vi "Test Engine Actor Register Events.vi"(8 "error in (no error)":errorcluster, 9 "Registrant Address":refnum<class "Message Enqueuer.lvclass">, 10 "Event Source Address":refnum<class "Message Enqueuer.lvclass">, 11 "TestBench in":refnum<class "TestBench.lvclass">) -> (0 "error out":errorcluster, 3 "TestBench out":refnum<class "TestBench.lvclass">)   [LabVIEW 2019, in "TestBench.lvlib" / "TestBench.lvclass"]
uses:
  TestBench.lvclass
  <vilib>/ActorFramework/Message Enqueuer/Message Enqueuer.lvclass
  TestEngine/TestEngine/TestEngineReference.lvclass
  C:/Program Files (x86)/National Instruments/LabVIEW 2019/vi.lib/NI/Event Source Actor/Event Source/Event/Event.lvclass
  TestBench Messages/Insert VI Msg/Insert VI Msg.lvclass
  C:/Program Files (x86)/National Instruments/LabVIEW 2019/vi.lib/NI/Event Source Actor/Event Source/Event Source Messages/Event Generated Msg/Event Generated Msg.lvclass
  TestBench Messages/Write DetailedResult Msg/Write DetailedResult Msg.lvclass
  TestEngine/TestEngine/TestResultInformation.lvclass
  TestBench Messages/Write TestResultInformation Msg/Write TestResultInformation Msg.lvclass
  TestEngine/TestEngine/Number of Steps.lvclass
  TestBench Messages/SetSlide Msg/SetSlide Msg.lvclass
  TestEngine/TestEngine/TestDetailedResult.lvclass
  TestBench Messages/StepCount Msg/StepCount Msg.lvclass
  <vilib>/NI/Event Source Actor/Event Source/Event/Event.lvclass/Event.ctl
  <vilib>/NI/Event Source Actor/Event Source/Event Source Messages/Register Msg/Register Msg.lvclass/Register Msg.ctl
  <vilib>/ActorFramework/Message Enqueuer/Message Enqueuer.lvclass/Message Enqueuer.ctl
  <vilib>/ActorFramework/Message Enqueuer/Enqueue.vi
  <vilib>/NI/Event Source Actor/Event Source/Event Source Messages/Register Msg/Register Msg.lvclass
  C:/Program Files (x86)/National Instruments/LabVIEW 2019/vi.lib/ActorFramework/Message/Message.lvclass
  <vilib>/ActorFramework/Message Priority Queue/Priority Enqueue.vi
  <vilib>/NI/Event Source Actor/Event Source/Event/Event.lvclass
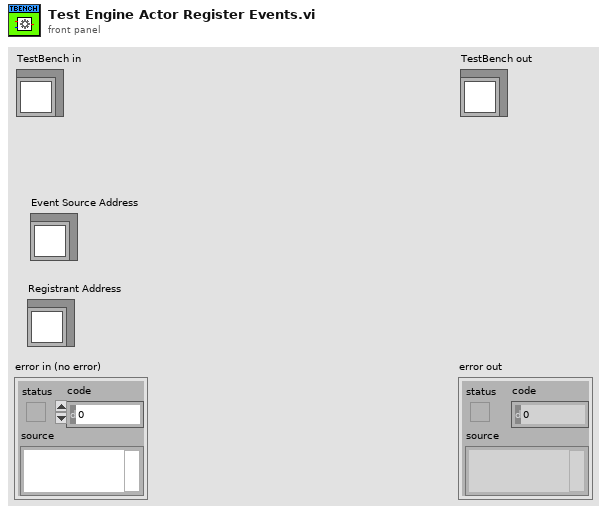
[diagram p1: front panel]
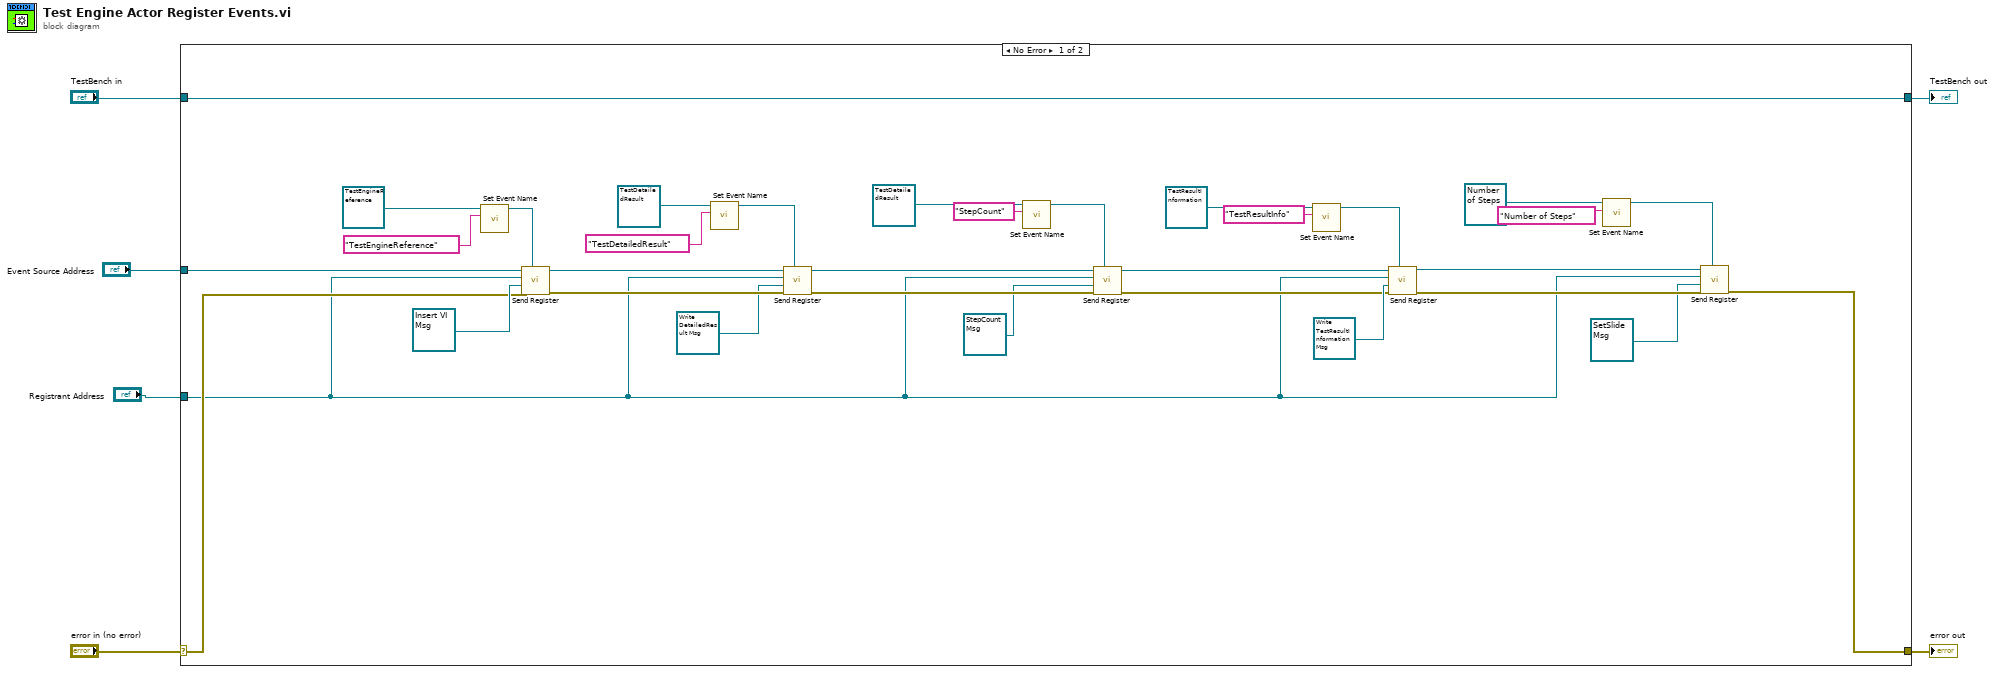
[diagram p0: block diagram]
diagram:
  n1 = case shown="No Error" "error in (no error)" {
    selector: "error in (no error)" -> [w10 w41]
    tunnel: [w7 w41] -> w5
    tunnel: [w39 w40] -> w3
    tunnel: "TestBench in" -> [w39 w40]
    tunnel: "Registrant Address" -> [w9 _]
    tunnel: "Event Source Address" -> [w8 _]
    frame No Error {
      n2 = call <vilib>:"Set Event Name.vi"("Name (Generic)"="TestEngineReference" ("ActorCoreEventMassage"), "Event In"=refnum<class "TestEngineReference.lvclass"> refnum ("TestEngine.lvlib:TestEngineReference.lvclass")) -> ("Event Out"=w37:refnum<class "TestEngineReference.lvclass">)  [unwired: 9 in]
      n3 = call <vilib>:"Send Register.vi"("Event"=w37, "Error In"=w10, "Event Handler"=refnum<class "Insert VI Msg.lvclass"> refnum ("TestBench.lvlib:Insert VI Msg.lvclass"), "Registrant Address"=w9, "Event Source Address"=w8) -> ("Error Out"=w30:errorcluster, "Event Source Address Out"=w31:refnum<class "Message Enqueuer.lvclass">)  [unwired: 5 in]
      n4 = call <vilib>:"Set Event Name.vi"("Name (Generic)"="TestDetailedResult", "Event In"=refnum<class "TestDetailedResult.lvclass"> refnum ("TestEngine.lvlib:TestDetailedResult.lvclass")) -> ("Event Out"=w32:refnum<class "TestDetailedResult.lvclass">)  [unwired: 9 in]
      n5 = call <vilib>:"Send Register.vi"("Event"=w32, "Error In"=w30, "Event Handler"=refnum<class "Write DetailedResult Msg.lvclass"> refnum ("TestBench.lvlib:Write DetailedResult Msg.lvclass"), "Registrant Address"=w9, "Event Source Address"=w31) -> ("Error Out"=w16:errorcluster, "Event Source Address Out"=w18:refnum<class "Message Enqueuer.lvclass">)  [unwired: 5 in]
      n6 = call <vilib>:"Set Event Name.vi"("Name (Generic)"="StepCount", "Event In"=refnum<class "TestDetailedResult.lvclass"> refnum ("TestEngine.lvlib:TestDetailedResult.lvclass")) -> ("Event Out"=w12:refnum<class "TestDetailedResult.lvclass">)  [unwired: 9 in]
      n7 = call <vilib>:"Send Register.vi"("Event"=w12, "Error In"=w16, "Event Handler"=refnum<class "StepCount Msg.lvclass"> refnum ("TestBench.lvlib:StepCount Msg.lvclass"), "Registrant Address"=w9, "Event Source Address"=w18) -> ("Error Out"=w15:errorcluster, "Event Source Address Out"=w17:refnum<class "Message Enqueuer.lvclass">)  [unwired: 5 in]
      n8 = call <vilib>:"Set Event Name.vi"("Name (Generic)"="TestResultInfo", "Event In"=refnum<class "TestResultInformation.lvclass"> refnum ("TestEngine.lvlib:TestResultInformation.lvclass")) -> ("Event Out"=w26:refnum<class "TestResultInformation.lvclass">)  [unwired: 9 in]
      n9 = call <vilib>:"Send Register.vi"("Event"=w26, "Error In"=w15, "Event Handler"=refnum<class "Write TestResultInformation Msg.lvclass"> refnum ("TestBench.lvlib:Write TestResultInformation Msg.lvclass"), "Registrant Address"=w9, "Event Source Address"=w17) -> ("Error Out"=w20:errorcluster, "Event Source Address Out"=w21:refnum<class "Message Enqueuer.lvclass">)  [unwired: 5 in]
      n10 = call <vilib>:"Set Event Name.vi"("Name (Generic)"="Number of Steps", "Event In"=refnum<class "Number of Steps.lvclass"> refnum ("TestEngine.lvlib:Number of Steps.lvclass")) -> ("Event Out"=w22:refnum<class "Number of Steps.lvclass">)  [unwired: 9 in]
      n11 = call <vilib>:"Send Register.vi"("Event"=w22, "Error In"=w20, "Event Handler"=refnum<class "SetSlide Msg.lvclass"> refnum ("TestBench.lvlib:SetSlide Msg.lvclass"), "Registrant Address"=w9, "Event Source Address"=w21) -> ("Error Out"=w7:errorcluster)  [unwired: 5 in, 1 out]
    }
    frame Error {
    }
  }
  "error out" <- w5
  "TestBench out" <- w3
